vi "Execute.vi"(8 "error in":errorcluster, 11 "Check Ozone Stability in":refnum<class "Check Ozone Stability.lvclass">) -> (0 "error out":errorcluster, 1 "Next Step?":bool, 2 "MSG":string, 3 "Check Ozone Stability out":refnum<class "Check Ozone Stability.lvclass">)   [LabVIEW 2013, in "Check Ozone Stability.lvclass"]
uses:
  Check Ozone Stability.lvclass
  Check Ozone Stability.lvclass/Check Ozone Stability.ctl
  Stability Step/Stability Step.lvclass/Stability Step.ctl
  Reusable/Sequence/STEPS/STEP.lvclass/STEP.ctl
  Read State DVR.vi
  Stability Step/Read # of Obs.vi
  Reusable/Sequence/STEPS/Read First Call.vi
  Stability Step/Read Error.vi
  Reusable/Sequence/STEPS/Write First Call.vi
  Reusable/PAS/Data/Main/Read CellData.vi
  Reusable/PAS/Data/Cell/Read derived.vi
  Data/cPAS Data.lvclass
  Reusable/PAS/Data/Cell/PAS Cell Data.lvclass
  <vilib>/Analysis/NI_AALBase.lvlib
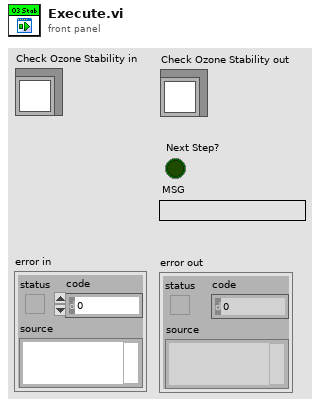
[diagram p1: front panel]
types:
  T1 = cluster{"f0":sgl, "IA":sgl, "Q":sgl, "max":dbl[], "deltaPhi":dbl, "tau":dbl, "noiseLim":dbl, "ext":dbl}
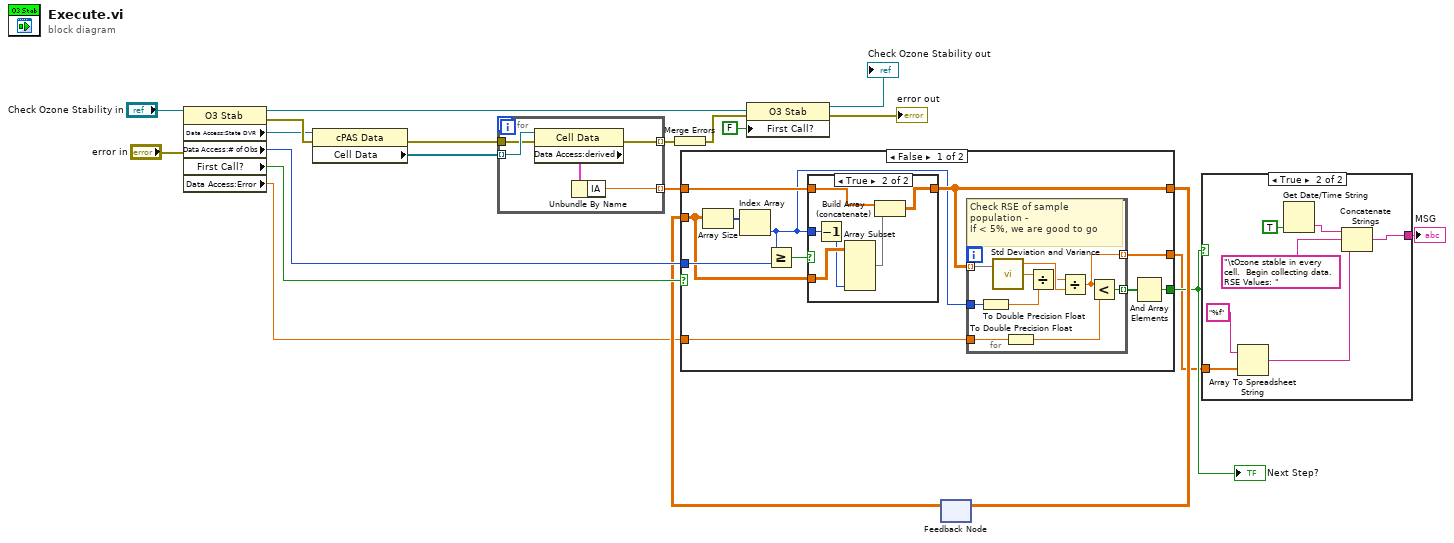
[diagram p0: block diagram]
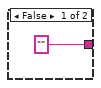
[diagram p2: hidden frame]
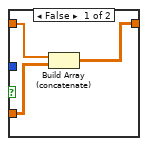
[diagram p3: hidden frame]
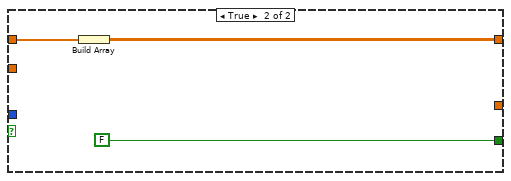
[diagram p4: hidden frame]
diagram:
  n1 = property class="O3 Stab"(reference="Check Ozone Stability in", error in="error in") -> (reference out=w19:refnum<class "Check Ozone Stability.lvclass">, error out=w8:errorcluster, "Data Access:State DVR"=w2:refnum<data-value>, "Data Access:# of Obs"=w16:u16, "First Call?"=w17:bool, "Data Access:Error"=w3:sgl)
  n2 = property class="cPAS Data"(reference=w2, error in=w8) -> (error out=w6:errorcluster, "Cell Data"=w20:refnum<class "PAS Cell Data.lvclass">[])  [unwired: 1 out]
  n3 = for {
    tunnel: w20 -> [w26] mode=indexing
    tunnel: [w24] -> w15 mode=indexing
    tunnel: w6 -> [w23]
    tunnel: [w22] -> w5 mode=indexing
    n4 = property class="Cell Data"(reference=w26, error in=w23) -> (error out=w22:errorcluster, "Data Access:derived"=w25:T1)  [unwired: 1 out]
    n5 = Unbundle By Name(w25) -> ("IA"=w24:sgl)
  }
  n6 = Merge Errors(w5) -> (w4:errorcluster)
  n7 = property class="O3 Stab"(reference=w19, error in=w4, "First Call?"=FALSE) -> (reference out=→"Check Ozone Stability out":refnum<class "Check Ozone Stability.lvclass">, error out=→"error out":errorcluster)
  n8 = feedback #1() -> (w13:sgl[][])  [unwired: 1 in]
  n9 = case shown="False" w17 {
    tunnel: w16 -> [w36 _]
    tunnel: w15 -> [w34 w59]
    tunnel: [w32 w58] -> w14
    tunnel: w13 -> [w33 _]
    tunnel: [w29 FALSE ("Boolean")] -> w10
    tunnel: w3 -> [w28 _]
    tunnel: [w27 _] -> w1
    frame False {
      n10 = Array Size(array=w33) -> (size(s)=w37:i32[])
      n11 = Index Array(array=w37) -> (element=w31:i32)  [unwired: 1 in]
      n12 = Greater Or Equal?(x=w31, y=w36) -> (x >= y?=w35:bool)
      n13 = case shown="True" w35 {
        tunnel: w34 -> [w50 w52]
        tunnel: w33 -> [w49 w55]
        tunnel: [w48 w51] -> w32
        tunnel: w31 -> [_ w56]
        frame False {
          n14 = Build Array (concatenate)(w50, w49) -> (w48:sgl[][])
        }
        frame True {
          n15 = Decrement(x=w56) -> (x-1=w54:i32)
          n16 = Array Subset(array=w55, length (col)=w54) -> (w53:sgl[][])  [unwired: 3 in]
          n17 = Build Array (concatenate)(w52, w53) -> (w51:sgl[][])
        }
      }
      n18 = for {
        tunnel: w32 -> [w47] mode=indexing
        tunnel: w31 -> [w42]
        tunnel: [w43] -> w30 mode=indexing
        tunnel: w28 -> [w40]
        tunnel: [w38] -> w27 mode=indexing
        # "Check RSE of sample population -\nIf < 5%, we are good to go"
        n19 = To Double Precision Float(number=w42) -> (double precision float=w41:dbl)
        n20 = call <vilib>:"Std Deviation and Variance.vi"("X"=w47) -> ("mean"=w45:dbl, "standard deviation"=w46:dbl)  [unwired: 1 in, 1 out]
        n21 = To Double Precision Float(number=w40) -> (double precision float=w39:dbl)
        n22 = Divide(x=w46, y=w41) -> (x/y=w44:dbl)
        n23 = Divide(x=w44, y=w45) -> (x/y=w38:dbl)
        n24 = Less?(x=w38, y=w39) -> (x < y?=w43:bool)
      }
      n25 = And Array Elements(Boolean array=w30) -> (logical AND=w29:bool)
    }
    frame True {
      n26 = Build Array(w59) -> (w58:sgl[][])
    }
  }
  "Next Step?" <- w10
  n27 = feedback-in #1(w14) -> ()
  n28 = case shown="True" w10 {
    tunnel: ["" w64] -> w9
    tunnel: w1 -> [_ w62]
    frame False {
    }
    frame True {
      n29 = Array To Spreadsheet String(array=w62, 3:"%f" ("format string")) -> (spreadsheet string=w61:string)  [unwired: 1 in]
      n30 = Get Date/Time String(want seconds? (F)=TRUE) -> (time string=w66:string)  [unwired: 2 in, 1 out]
      n31 = Concatenate Strings(w66, "\tOzone stable in every cell.  Begin collecting data. RSE Values: " ("string"), w61) -> (w64:string)
    }
  }
  "MSG" <- w9
